vi "FOFB Data Archiver Main.vi"() -> ()   [LabVIEW 2011]
uses:
  Types Definitions/Type BPM and PS select cluster.ctl
  <vilib>/Platform/TimedLoop/XDataNode/timing_clust.ctl
  <vilib>/Platform/TimedLoop/XDataNode/nitl_modes.ctl
  <vilib>/Platform/TimedLoop/XDataNode/wakeup.ctl
  <vilib>/Platform/TimedLoop/XDataNode/XDataNode.xnode
  Type Definitions.lvlib
  <vilib>/Platform/TimedLoop/XDataNode/XDNodeRunTimeDep.lvlib
  File VIs.lvlib
  kernel32.dll
  <vilib>/addons/internet/NI_InternetTK_FTP_VIs.lvlib
  Controller VIs.lvlib
panel:
  out "Slide":dbl(slide)
  out "Next filename":string caption="Registro de dados em:"
  out "Status":bool caption="Registrando dados..."
  in  "Path":path=path "E:/" caption="Diretório de armazenamento"
  in  "Maximum number of files":i32=18900 caption="Máximo número de arquivos:"
  in  "Number of packets per file":i32=1000 caption="Número de pacotes de dados por arquivo:"
  in  "FOFB Controller IP":string="10.0.5.31" caption="IP do controlador do FOFB (PXI):"
  in  "stop":bool
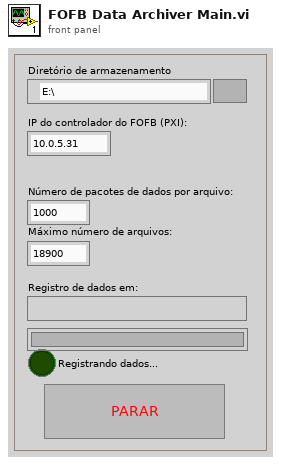
[diagram p1: front panel]
types:
  T1 = typedef "Type Definitions.lvlib/Type BPM and PS select cluster.ctl" = cluster{"BPM index array":u32[], "PS index array ":u32[]}
  T2 = enum16{"Idle", "Wait Connection", "Read Data", "Close Connection"}
  T3 = typedef "XDNodeRunTimeDep.lvlib/timing_clust.ctl" = cluster{"Expected End [f-1]":u64, "Actual End [f-1]":u64, "Finished Late? [f-1]":bool, "Expected End [i-1]":u64, "Actual End [i-1]":u64, "Finished Late? [i-1]":bool, "Expected Start [i]":u64, "Actual Start [i]":u64, "Expected Start [f]":u64, "Actual Start [f]":u64, "Source Name":string, "Structure Name":string, "Period":i64, "Deadline":i64, "Offset":i64, "Start":i64, "Priority":i32, "Timeout":i32, "Mode":T4, "Wakeup Reason":T5, "Error":errorcluster, "Source Type":string, "Secondary Source Type":string, "Global End Time":u64, "Global Start Time":u64, "Frame Duration":u64, "Iteration Duration":u64, "Assigned CPU":i32, "I/O Scan Engine Mode":u32}
  T4 = typedef "XDNodeRunTimeDep.lvlib/nitl_modes.ctl" = enum32{"No Change", "Process missed periods, maintain original phase", "Discard missed periods, maintain original phase", "Process missed periods, ignore original phase", "Discard missed periods, ignore original phase"}
  T5 = typedef "XDNodeRunTimeDep.lvlib/wakeup.ctl" = enum32{"Normal", "Aborted", "Asynchronous wakeup", "Timing source error", "Timed loop error", "Timeout"}
  T6 = enum16{"open", "replace", "create", "open or create", "replace or create", "replace or create with confirmation"}
  T7 = typedef "Type Definitions.lvlib/Type FOFB Configuration.ctl" = cluster{"FOFB Parameters":T8, "Number of Acquisition Chassis":i32, "Number of Actuation Chassis":i32, "Number of BPM Readings":i32, "BPM Reading Names":string[], "Selected BPM Readings":u32[], "Number of Correctors":i32, "Corrector Names":string[], "Selected Correctors":u32[], "Response Matrix":dbl[][][], "Reference Orbit":dbl[][], "Correction Matrix":dbl[][][], "FPGA Filter Sets":cluster{"BPM Filter Coefficients":dbl[][], "PS Filter Coefficients":dbl[][]}[], "Acquisition Chassis Names":string[], "Actuation Chassis Names":string[], "Acquisition Variables":cluster{"Variable Name":string, "Chassis Name":string}[], "Actuation Variables":cluster{"Variable Name":string, "Chassis Name":string}[], "PS Matrix Mapping":cluster{u32[]}[], "Inverse PS Matrix Mapping":u32[][], "BPM Matrix Mapping":cluster{u32[]}[], "Inverse BPM Matrix Mapping":u32[][], "BPM Planes":enum8{"H", "V"}[], "Corrector Planes":enum8{"H", "V"}[]}
  T8 = typedef "Type Definitions.lvlib/Type FOFB Parameters.ctl" = cluster{"Network":T9, "Fast Acquisition":T10, "Acquisition Network":T11, "Actuation Network":T12}
  T9 = typedef "Type Definitions.lvlib/Type Network Configuration.ctl" = cluster{"FOFB Controller IP":string, "LNLS Control Network IP":string, "LNLS Control Network Power Supplies TCP Port":u16, "LNLS Control Network FOFB Configuration TCP Port":u16, "LNLS Control Network BPMs TCP Port":u16, "Monitoring Data TCP Port":u16, "Fast Archiver TCP Port":u16, "Fast Command TCP Port":u16, "TCP Listening Timeout":i32}
  T10 = typedef "Type Definitions.lvlib/Type FA Configuration.ctl" = cluster{"Sampling Period":u32, "Data Buffer Size":u32, "Monitoring Period":u32}
  T11 = typedef "Type Definitions.lvlib/Type Acquisition Network Configuration.ctl" = cluster{"Chassis Name":string, "Variables":cluster{"Variable Name":string, "Matrix Order":u32, "Plane":enum8{"H", "V"}, "On Correction":bool}[]}[]
  T12 = typedef "Type Definitions.lvlib/Type Actuation Network Configuration.ctl" = cluster{"Chassis Name":string, "Variables":cluster{"Variable Name":string, "Matrix Order":u32, "Plane":enum8{"H", "V"}, "On Correction":bool}[]}[]
  T13 = enum16{"Standard", "Buffered", "CRLF", "Immediate"}
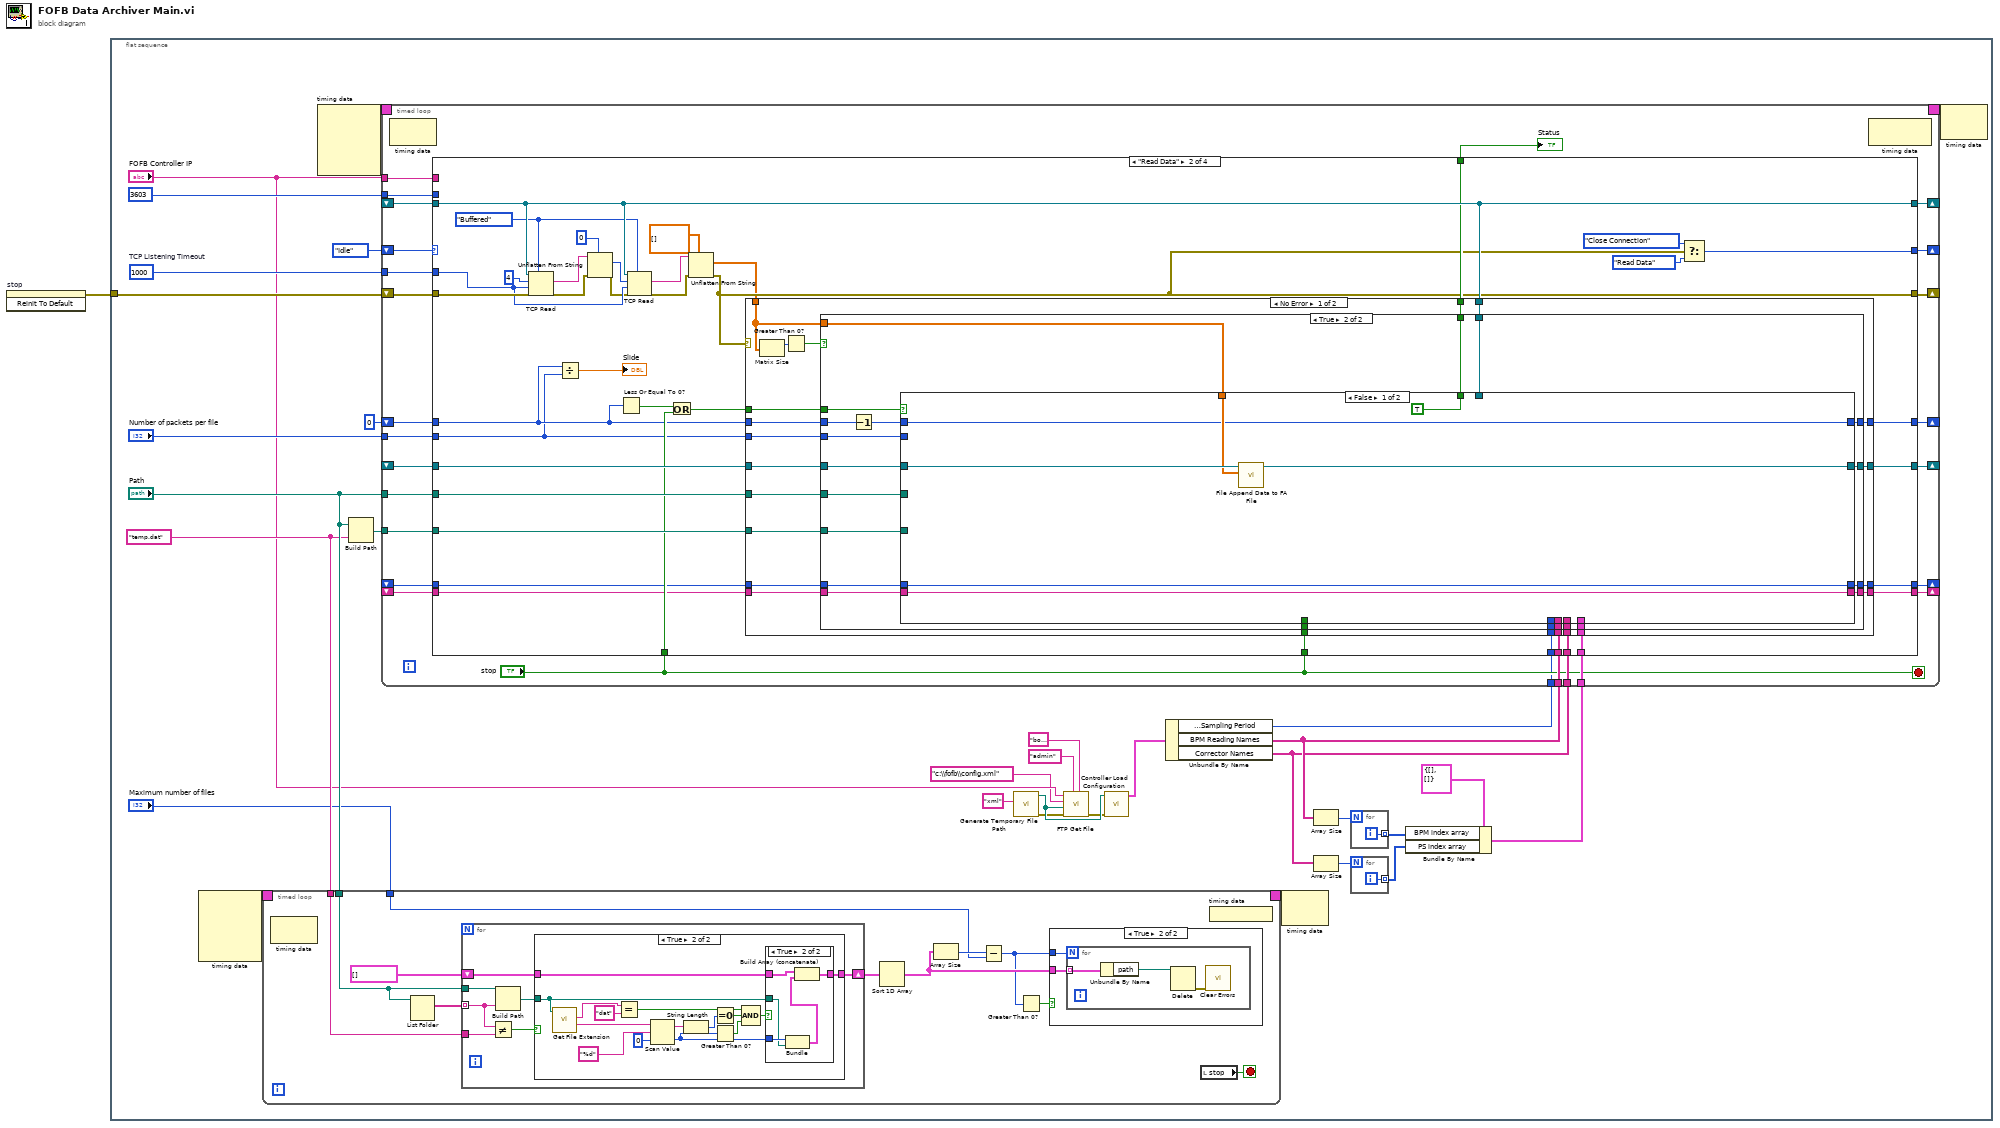
[diagram p0: block diagram]
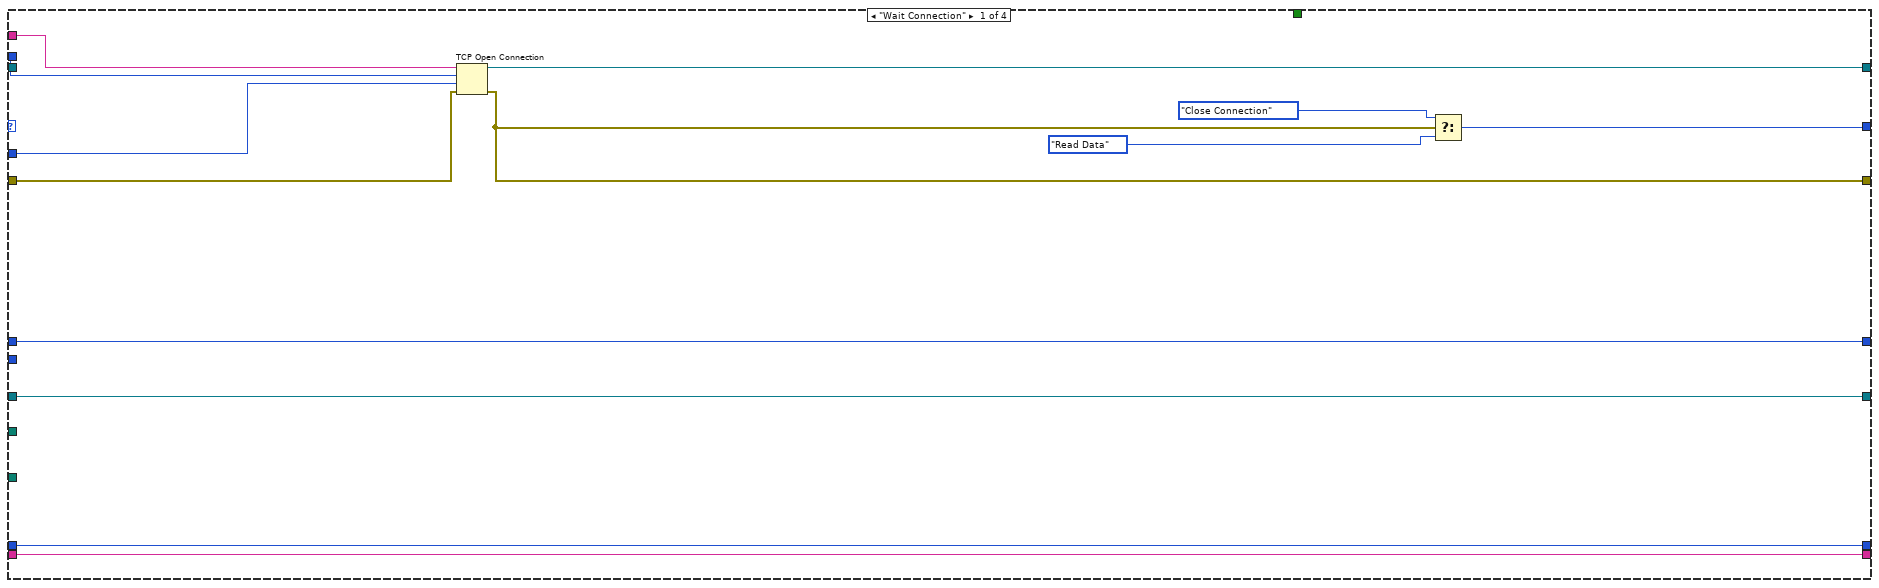
[diagram p2: hidden frame]
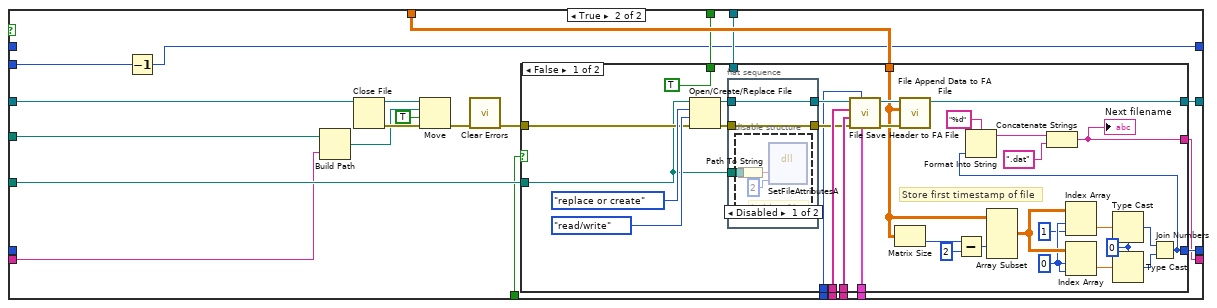
[diagram p4: hidden frame]
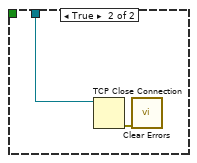
[diagram p6: hidden frame]
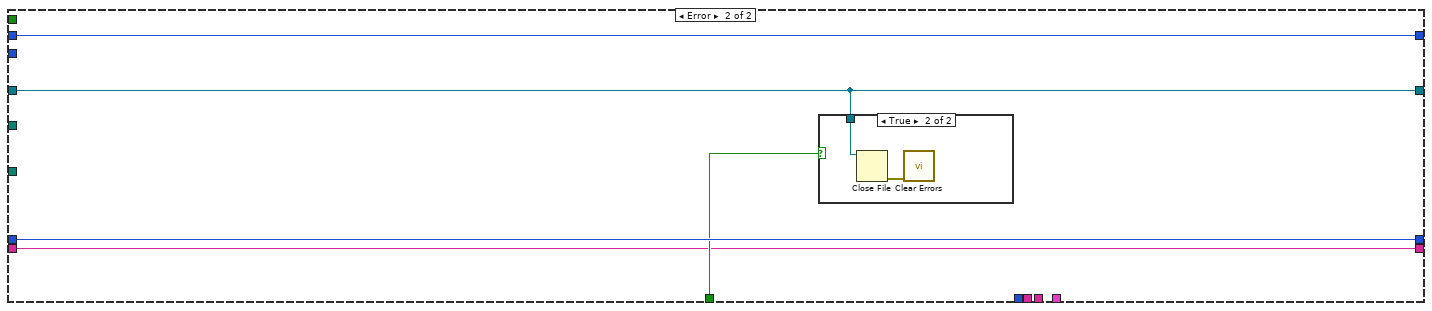
[diagram p7: hidden frame]
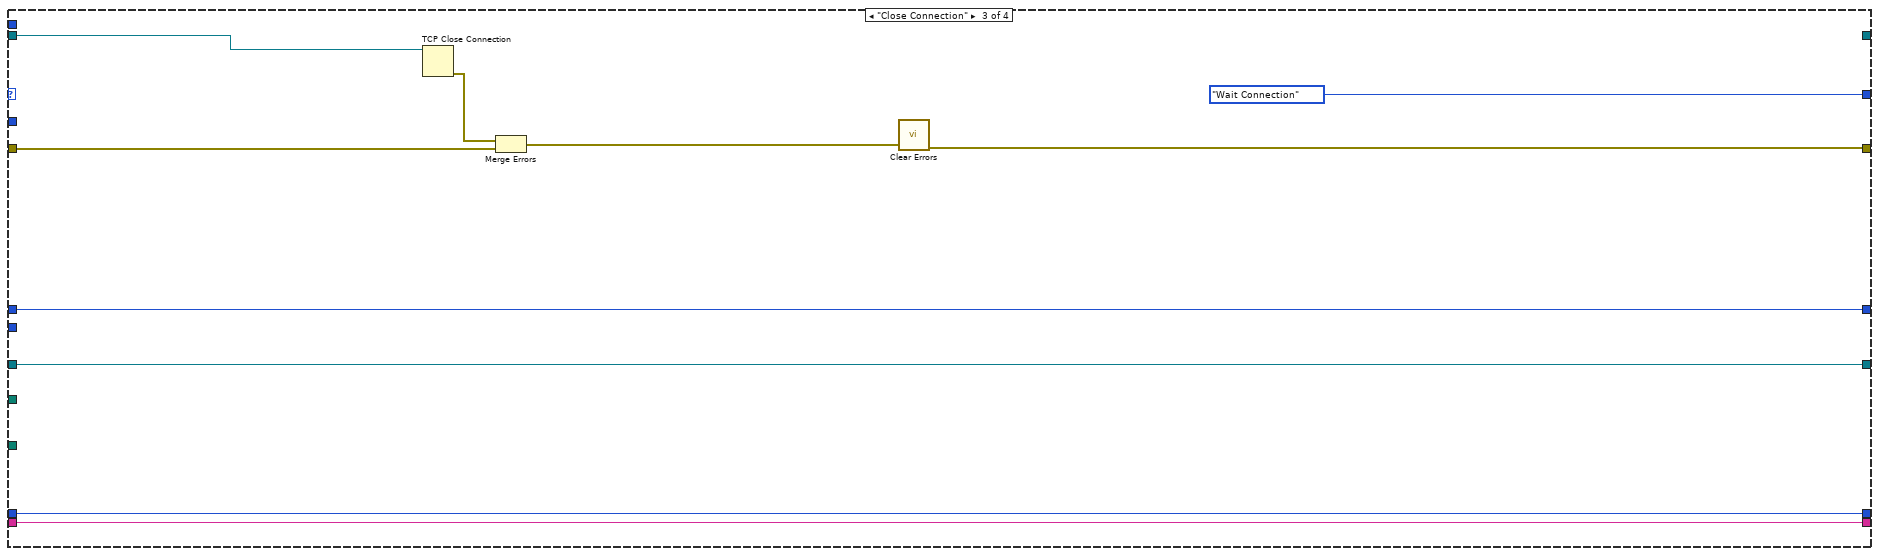
[diagram p9: hidden frame]
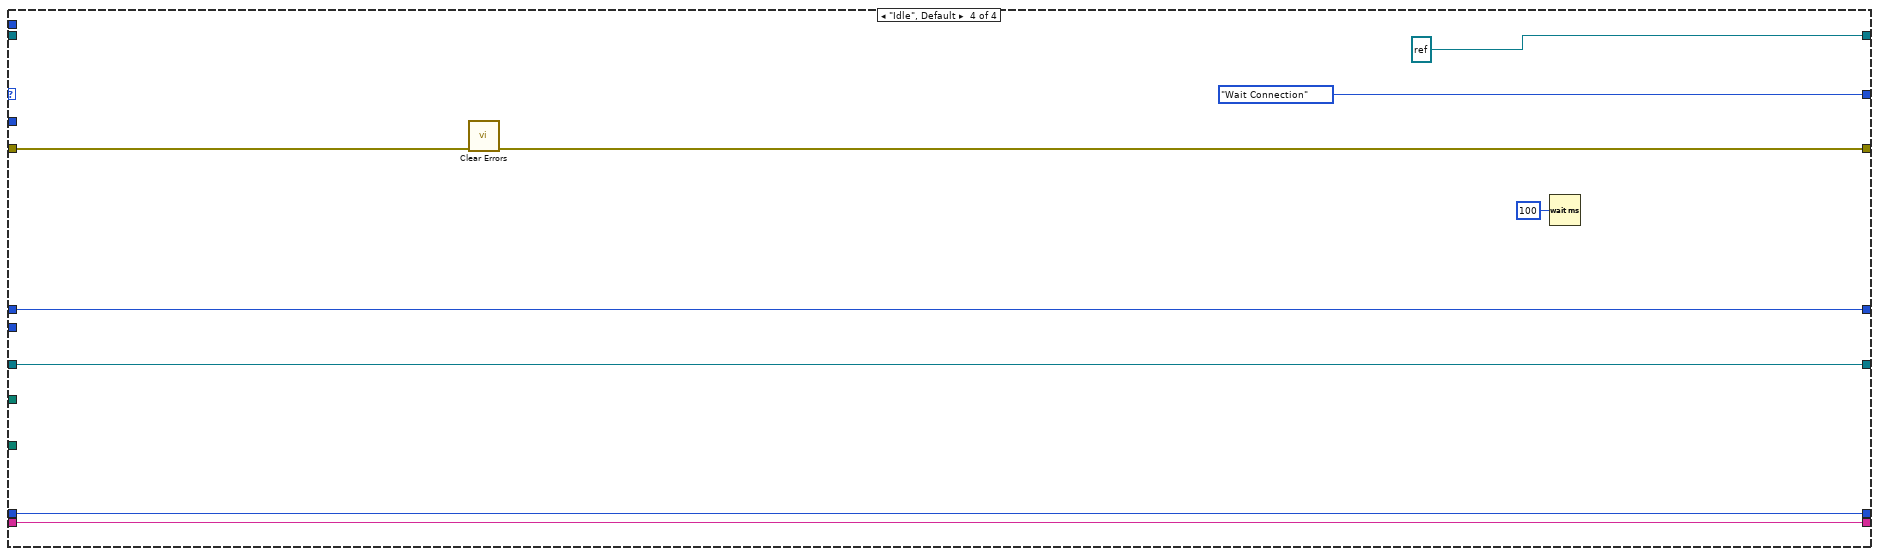
[diagram p10: hidden frame]
diagram:
  n1 = invoke on="stop" class="Bool (strict)" method="Reinit To Default"() -> (error out=w1:errorcluster)  [unwired: 3 in, 2 out]
  n2 = flat-sequence {
    tunnel: w1 -> [w16]
    frame #0 {
      w18 = "temp.dat" ("FOFB Controller IP")
      w22 = 1000  # TCP Listening Timeout
      n3 = node-c288() -> (w33:T3)  [unwired: 4 in]
      n4 = timed-loop {
        timing: w33 -> [_]
        timing-out: [_] -> w32
        tunnel: "Path" -> [w263]
        tunnel: w18 -> [w265]
        tunnel: "Maximum number of files" -> [w264]
        stop <- w266 stop-if-true
        n5 = node-c288() -> ()  [unwired: 1 in, 1 out]
        n6 = List Folder(path=w263) -> (filenames=w270:string[])  [unwired: 3 in, 3 out]
        n7 = for {
          tunnel: w263 -> [w282]
          tunnel: w270 -> [w277] mode=indexing
          shift-right: [w281] -> w268
          shift-left: cluster{"timestamp":u64, "path":path}[] [] -> [w279]
          tunnel: w265 -> [w276]
          n8 = Not Equal?(x=w277, y=w276) -> (x != y?=w278:bool)
          n9 = Build Path(base path=w282, name or relative path=w277) -> (appended path=w280:path)
          n10 = case shown="True" w278 {
            tunnel: [w283 w298] -> w281
            tunnel: w280 -> [_ w295]
            tunnel: w279 -> [w283 w297]
            frame False {
            }
            frame True {
              n11 = call <vilib>:"Get File Extension.vi"("file"=w295) -> ("filename without extension"=w293:string, "lowercase file extension"=w294:string)  [unwired: 7 in, 2 out]
              n12 = Equal?(x=w294, y="dat") -> (x = y?=w291:bool)
              n13 = Scan Value(string=w293, format string="%d", default (0 dbl)=u64 0 ("const")) -> (output string=w284:string, value=w288:u64)
              n14 = String Length(string=w284) -> (length=w285:i32)
              n15 = Equal To 0?(x=w285) -> (x = 0?=w286:bool)
              n16 = Greater Than 0?(x=w288) -> (x > 0?=w287:bool)
              n17 = Compound Arithmetic op=AND(w291, w286, w287) -> (w290:bool)
              n18 = case shown="True" w290 {
                tunnel: w297 -> [w299 w304]
                tunnel: [w299 w303] -> w298
                tunnel: w295 -> [_ w300]
                tunnel: w288 -> [_ w301]
                frame False {
                }
                frame True {
                  n19 = Bundle("const"=w301, "appended path"=w300) -> (w302:cluster{"const":u64, "appended path":path})  [unwired: 1 in]
                  n20 = Build Array (concatenate)(w304, w302) -> (w303:cluster{"const":u64, "appended path":path}[])
                }
              }
            }
          }
        }
        n21 = Sort 1D Array(array=w268) -> (sorted array=w262:cluster{"timestamp":u64, "path":path}[])
        n22 = Array Size(array=w262) -> (size(s)=w267:i32)
        n23 = Subtract(x=w267, y=w264) -> (x-y=w261:i32)
        n24 = Greater Than 0?(x=w261) -> (x > 0?=w260:bool)
        n25 = case shown="True" w260 {
          tunnel: w262 -> [_ w271]
          tunnel: w261 -> [_ w272]
          frame False {
          }
          frame True {
            n26 = for {
              N: w272 -> [_]
              tunnel: w271 -> [w275] mode=indexing
              n27 = Unbundle By Name(w275) -> ("path"=w274:path)
              n28 = Delete(path (use dialog)=w274) -> (error out=w273:errorcluster)  [unwired: 4 in, 2 out]
              n29 = call <vilib>:"Clear Errors.vi"("error in (no error)"=w273) -> ()  [unwired: 6 in, 1 out]
            }
          }
        }
        n30 = local read "stop"() -> (w266:bool)
        n31 = node-c288() -> ()  [unwired: 1 out]
      }
      n32 = node-c288() -> (w12:T3)  [unwired: 4 in]
      n33 = Build Path(base path="Path", name or relative path=w18) -> (appended path=w29:path)
      n34 = call <vilib>:"Generate Temporary File Path.vi"("Temporary File Extension (tmp)"="xml") -> ("error out"=w2:errorcluster, "Unique Temporary File Path"=w5:path)  [unwired: 9 in]
      n35 = call <vilib>:"FTP Get File.vi"("password"="boo500mev", "user"="admin", "error in (no error)"=w2, "local path"=w5, "remote path"="c:\\fofb\\config.xml", "host"="FOFB Controller IP") -> ("error out"=w3:errorcluster)  [unwired: 4 in, 1 out]
      n36 = call "Controller Load Configuration.vi"("error in (no error)"=w3, "FOFB Configuration Path"=w5) -> ("FOFB Configuration"=w4:T7)  [unwired: 8 in, 1 out]
      n37 = Unbundle By Name(w4) -> ("FOFB Parameters.Fast Acquisition.Sampling Period"=w15:u32, "BPM Reading Names"=w21:string[], "Corrector Names"=w20:string[])
      n38 = node-c288(w32) -> ()  [unwired: 1 out]
      n39 = Array Size(array=w21) -> (size(s)=w28:i32)
      n40 = Array Size(array=w20) -> (size(s)=w24:i32)
      n41 = for {
        N: w28 -> [_]
        tunnel: [w310] -> w25 mode=indexing
        i -> [w310]
      }
      n42 = for {
        N: w24 -> [_]
        tunnel: [w309] -> w23 mode=indexing
        i -> [w309]
      }
      n43 = Bundle By Name(cluster=T1 {"BPM index array"=[], "PS index array "=[]} ("BPM and PS selection"), "BPM index array"=w25, "PS index array"=w23) -> (w27:T1)
      n44 = timed-loop {
        shift-right: [w51] -> _
        shift-left: w16 -> [w59]
        shift-right: [w55] -> _
        shift-left: T2."Idle" ("f") -> [w57]
        shift-right: [w56] -> _
        shift-left: _ -> [w58]
        tunnel: "FOFB Controller IP" -> [w54]
        tunnel: u16 3603 ("TCP Port") -> [w53]
        tunnel: w22 -> [w52]
        shift-right: [w49] -> _
        shift-left: 0 ("Number of packets per file") -> [w50]
        tunnel: "Number of packets per file" -> [w48]
        shift-right: [w47] -> _
        shift-left: _ -> [w46]
        tunnel: w29 -> [w45]
        tunnel: "Path" -> [w44]
        tunnel: w21 -> [w43]
        tunnel: w20 -> [w42]
        tunnel: w27 -> [w41]
        tunnel: w15 -> [w38]
        shift-right: [w36] -> _
        shift-left: _ -> [w37]
        shift-right: [w35] -> _
        shift-left: _ -> [w34]
        timing: w12 -> [_]
        timing-out: [_] -> w11
        stop <- "stop" stop-if-true
        n45 = node-c288() -> ()  [unwired: 1 in, 1 out]
        n46 = case shown="\"Read Data\"" w57 {
          tunnel: [w74 w90 _ refnum<k5> refnum ("connection ID")] -> w56
          tunnel: [w73 w113 T2."Wait Connection" ("f") T2."Wait Connection" ("f")] -> w55
          tunnel: [w67 w83 w243 w254] -> w51
          tunnel: w59 -> [w72 w112 w245 w255]
          tunnel: w58 -> [_ w90 w248 _]
          tunnel: w54 -> [w69 _ _ _]
          tunnel: w53 -> [w68 _ _ _]
          tunnel: w52 -> [w66 w103 _ _]
          tunnel: w50 -> [w63 w77 w240 w250]
          tunnel: [w63 w102 w240 w250] -> w49
          tunnel: w48 -> [_ w76 _ _]
          tunnel: [w65 w101 w242 w252] -> w47
          tunnel: w46 -> [w65 w100 w242 w252]
          tunnel: w45 -> [_ w99 _ _]
          tunnel: w44 -> [_ w98 _ _]
          tunnel: "stop" -> [_ w97 _ _]
          tunnel: "stop" -> [_ w94 _ _]
          tunnel: w43 -> [_ w93 _ _]
          tunnel: w42 -> [_ w92 _ _]
          tunnel: w41 -> [_ w91 _ _]
          tunnel: [_ w89 _ _] -> w39
          tunnel: w38 -> [_ w88 _ _]
          tunnel: w37 -> [w64 w82 w241 w251]
          tunnel: [w64 w87 w241 w251] -> w36
          tunnel: [w62 w80 w239 w249] -> w35
          tunnel: w34 -> [w62 w79 w239 w249]
          frame "Wait Connection" {
            n47 = TCP Open Connection(address=w69, remote port or service name=w68, timeout ms (60000)=w66, error in (no error)=w72) -> (connection ID=w74:refnum<k5>, error out=w67:errorcluster)  [unwired: 1 in]
            n48 = Select(t=T2."Close Connection" ("f"), s=w67, f=T2."Read Data") -> (s? t:f=w73:T2)
          }
          frame "Read Data" {
            w81 = T13."Buffered" ("mode (standard)")
            n49 = TCP Read(connection ID=w90, bytes to read=4, error in (no error)=w112, 7:w81, 9:w103) -> (data out=w108:string, error out=w86:errorcluster)  [unwired: 1 out]
            n50 = Divide(x=w77, y=w76) -> (x/y=→"Slide":dbl)
            n51 = Unflatten From String(type=0 ("bytes to read"), binary string=w108, error in (no error)=w86) -> (value=w106:i32, error out=w85:errorcluster)  [unwired: 2 in, 1 out]
            n52 = Less Or Equal To 0?(x=w77) -> (x <= 0?=w95:bool)
            n53 = TCP Read(connection ID=w90, bytes to read=w106, error in (no error)=w85, 7:w81, 9:w103) -> (data out=w105:string, error out=w84:errorcluster)  [unwired: 1 out]
            n54 = Or(x=w95, y=w97) -> (x .or. y?=w96:bool)
            n55 = Unflatten From String(type=sgl[][] [] ("BPM and PS Data"), binary string=w105, error in (no error)=w84) -> (value=w75:sgl[][], error out=w83:errorcluster)  [unwired: 2 in, 1 out]
            n56 = case shown="No Error" w83 {
              tunnel: [w135 w236] -> w102
              tunnel: w76 -> [w134 _]
              tunnel: w77 -> [w117 w236]
              tunnel: w75 -> [w119 _]
              tunnel: [w133 w233] -> w101
              tunnel: w100 -> [w132 w233]
              tunnel: w99 -> [w131 _]
              tunnel: w98 -> [w130 _]
              tunnel: w96 -> [w129 _]
              tunnel: w94 -> [w128 w234]
              tunnel: w93 -> [w127 _]
              tunnel: w92 -> [w126 _]
              tunnel: w91 -> [w125 _]
              tunnel: w90 -> [w124 _]
              tunnel: [w123 _] -> w89
              tunnel: w88 -> [w122 _]
              tunnel: w82 -> [w121 w235]
              tunnel: [w120 w235] -> w87
              tunnel: [w115 w232] -> w80
              tunnel: w79 -> [w114 w232]
              frame No Error {
                n57 = Matrix Size(0:w119) -> (1:w118:i32)  [unwired: 1 out]
                n58 = Greater Than 0?(x=w118) -> (x > 0?=w116:bool)
                n59 = case shown="True" w116 {
                  tunnel: [w137 w145] -> w135
                  tunnel: w134 -> [_ w160]
                  tunnel: w117 -> [w137 w144]
                  tunnel: [w139 w159] -> w133
                  tunnel: w132 -> [w139 w158]
                  tunnel: w131 -> [_ w157]
                  tunnel: w130 -> [_ w156]
                  tunnel: w129 -> [_ w143]
                  tunnel: w128 -> [_ w155]
                  tunnel: w127 -> [_ w154]
                  tunnel: w126 -> [_ w153]
                  tunnel: w125 -> [_ w152]
                  tunnel: w124 -> [_ w151]
                  tunnel: [_ w150] -> w123
                  tunnel: w122 -> [_ w149]
                  tunnel: w121 -> [w138 w148]
                  tunnel: [w138 w147] -> w120
                  tunnel: w119 -> [_ w146]
                  tunnel: [w136 w142] -> w115
                  tunnel: w114 -> [w136 w141]
                  frame False {
                  }
                  frame True {
                    n60 = Decrement(x=w144) -> (x-1=w140:i32)
                    n61 = case shown="False" w143 {
                      tunnel: [w162 w170] -> w145
                      tunnel: w160 -> [_ w171]
                      tunnel: w146 -> [w163 w181]
                      tunnel: [w167 w183] -> w159
                      tunnel: w158 -> [w166 w190]
                      tunnel: w157 -> [_ w189]
                      tunnel: w156 -> [_ w188]
                      tunnel: w148 -> [w165 _]
                      tunnel: [w165 w180] -> w147
                      tunnel: w155 -> [_ w179]
                      tunnel: w154 -> [_ w178]
                      tunnel: w153 -> [_ w177]
                      tunnel: w152 -> [_ w176]
                      tunnel: w151 -> [_ w175]
                      tunnel: [TRUE ("stop 2") w174] -> w150
                      tunnel: w149 -> [_ w173]
                      tunnel: w140 -> [w162 _]
                      tunnel: [w161 w169] -> w142
                      tunnel: w141 -> [w161 w168]
                      frame False {
                        n62 = call "File Append Data to FA File.vi"("Data"=w163, "FA File Reference"=w166) -> ("FA File Reference"=w167:refnum<file>)  [unwired: 7 in, 1 out]
                      }
                      frame True {
                        n63 = Decrement(x=w171) -> (x-1=w170:i32)
                        n64 = Build Path(base path=w188, name or relative path=w168) -> (appended path=w185:path)
                        n65 = Close File(refnum=w190) -> (path=w186:path, error out=w187:errorcluster)  [unwired: 1 in]
                        n66 = Move(source path=w186, error in=w187, 9:TRUE ("overwrite (F)"), 10:w185) -> (error out=w172:errorcluster)  [unwired: 1 in, 2 out]
                        n67 = call <vilib>:"Clear Errors.vi"("error in (no error)"=w172) -> ("error out"=w182:errorcluster)  [unwired: 6 in]
                        n68 = case shown="False" w179 {
                          tunnel: w189 -> [w212 _]
                          tunnel: [w221 _] -> w183
                          tunnel: w182 -> [w218 _]
                          tunnel: w181 -> [w217 _]
                          tunnel: [w192 _] -> w180
                          tunnel: w178 -> [w215 _]
                          tunnel: w177 -> [w214 _]
                          tunnel: w176 -> [w213 _]
                          tunnel: w175 -> [_ w231]
                          tunnel: [TRUE ("stop 2") _] -> w174
                          tunnel: w173 -> [w206 _]
                          tunnel: [w191 _] -> w169
                          frame False {
                            w203 = u32 0
                            w197 = 0 ("row 1")
                            # "Store first timestamp of file"
                            n69 = Open/Create/Replace File(file path (use dialog)=w212, error in=w218, operation (0:open)=T6."replace or create", access (0:read/write)=enum16{"read/write", "read-only", "write-only"}."read/write") -> (refnum out=w208:refnum<file>, error out=w210:errorcluster)  [unwired: 2 in, 1 out]
                            n70 = flat-sequence {
                              tunnel: w212 -> [w226]
                              tunnel: [w225] -> w211
                              tunnel: w210 -> [w225]
                              tunnel: [w224] -> w209
                              tunnel: w208 -> [w224]
                              frame #0 {
                                n71 = disable-structure shown="Disabled" {
                                disable-tunnel: w226 -> [w228 _]
                                frame Disabled {
                                # "hidden file"
                                n72 = Path To String(path=w228) -> (string=w227:string)
                                n73 = dll-call lib="kernel32.dll" fn="SetFileAttributesA"("lpFileName"=w227, "dwFileAttributes"=u32 2) -> ()  [unwired: 6 in, 2 out]
                                }
                                frame Enabled {
                                }
                                }
                              }
                            }
                            n74 = call "File Save Header to FA File.vi"("BPM and PS selection"=w213, "Acquisition period (us)"=w206, "error in (no error)"=w211, "PS Reading Names"=w214, "BPM Reading Names"=w215, "FA File Reference"=w209) -> ("error out"=w220:errorcluster, "FA File Reference out"=w219:refnum<file>)  [unwired: 4 in]
                            n75 = Matrix Size(0:w217) -> (2:w205:i32)  [unwired: 1 out]
                            n76 = call "File Append Data to FA File.vi"("error in (no error)"=w220, "Data"=w217, "FA File Reference"=w219) -> ("FA File Reference"=w221:refnum<file>)  [unwired: 6 in, 1 out]
                            n77 = Subtract(x=w205, y=2) -> (x-y=w216:i32)
                            n78 = Array Subset(array=w217, index (col)=w216) -> (w201:sgl[][])  [unwired: 3 in]
                            n79 = Index Array(array=w201, index (row)=w197, index (col)=1) -> (element=w200:sgl)
                            n80 = Index Array(array=w201, index (row)=w197, index (col)=w197) -> (element=w202:sgl)
                            n81 = Type Cast(type=w203, x=w200) -> (*(type *) &x=w199:u32)
                            n82 = Type Cast(type=w203, x=w202) -> (*(type *) &x=w198:u32)
                            n83 = Join Numbers(hi=w199, lo=w198) -> ((hi.lo)=w192:u64)
                            n84 = Format Into String(format string="%d", w192) -> (resulting string=w195:string)  [unwired: 2 in, 1 out]
                            n85 = Concatenate Strings(w195, ".dat" ("time format string (%c)")) -> (w191:string)
                            "Next filename" <- w191
                          }
                          frame True {
                            n86 = TCP Close Connection(connection ID=w231) -> (error out=w230:errorcluster)  [unwired: 2 in, 1 out]
                            n87 = call <vilib>:"Clear Errors.vi"("error in (no error)"=w230) -> ()  [unwired: 6 in, 1 out]
                          }
                        }
                      }
                    }
                  }
                }
              }
              frame Error {
                n88 = case shown="True" w234 {
                  tunnel: w233 -> [_ w238]
                  frame False {
                  }
                  frame True {
                    n89 = Close File(refnum=w238) -> (error out=w237:errorcluster)  [unwired: 1 in, 1 out]
                    n90 = call <vilib>:"Clear Errors.vi"("error in (no error)"=w237) -> ()  [unwired: 6 in, 1 out]
                  }
                }
              }
            }
            n91 = Select(t=T2."Close Connection" ("f"), s=w83, f=T2."Read Data") -> (s? t:f=w113:T2)
          }
          frame "Close Connection" {
            n92 = TCP Close Connection(connection ID=w248) -> (error out=w246:errorcluster)  [unwired: 2 in, 1 out]
            n93 = Merge Errors(w246, w245) -> (w244:errorcluster)
            n94 = call <vilib>:"Clear Errors.vi"("error in (no error)"=w244) -> ("error out"=w243:errorcluster)  [unwired: 6 in]
          }
          frame "Idle", Default {
            n95 = call <vilib>:"Clear Errors.vi"("error in (no error)"=w255) -> ("error out"=w254:errorcluster)  [unwired: 6 in]
            n96 = Wait (ms)(milliseconds to wait=u32 100 ("millisecond multiple")) -> ()  [unwired: 1 out]
          }
        }
        "Status" <- w39
        n97 = node-c288() -> ()  [unwired: 1 in, 1 out]
      }
      n98 = node-c288(w11) -> ()  [unwired: 1 out]
    }
  }
